vi "Break down String.vi"(6 "PlayerID":u8=1, 8 "Error in":errorcluster, 11 "Input String":string) -> (0 "Error Out":errorcluster, 3 "Output":string[](array[string]))   [LabVIEW 2018, in "Vires VTD System Explorer.lvlib"]
uses:
  Vires VTD System Explorer.lvlib
  <vilib>/regexp/Match Regular Expression.xnode
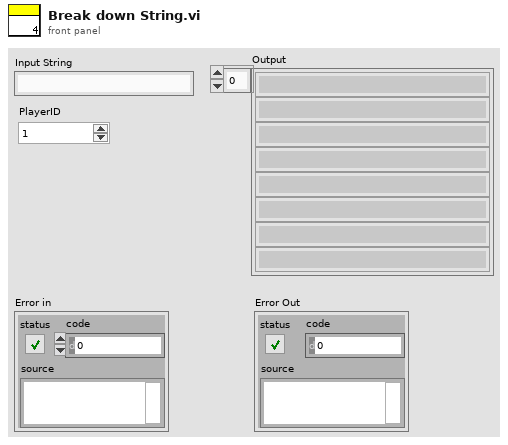
[diagram p1: front panel]
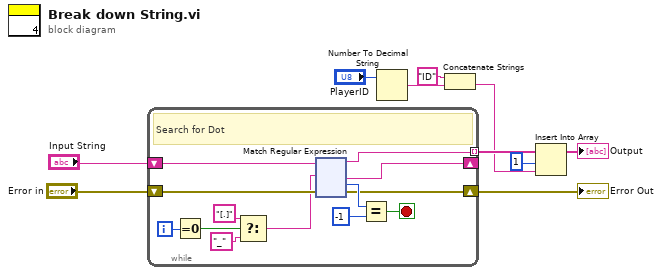
[diagram p0: block diagram]
diagram:
  n1 = while {
    shift-right: [w22] -> _
    shift-left: "Input String" -> [w23]
    tunnel: [w21] -> w4 mode=indexing
    shift-right: [w16] -> w8
    shift-left: "Error in" -> [w17]
    i -> [w15]
    stop <- w18 stop-if-true
    # "Search for Dot"
    n2 = Equal To 0?(x=w15) -> (x = 0?=w14:bool)
    n3 = Select(t="[.]" ("regular expression"), s=w14, f="_" ("regular expression")) -> (s? t:f=w11:string)
    n4 = xnode "Match Regular Expression"("input string"=w23, "regular expression"=w11, "error in"=w17) -> ("before match"=w21:string, "after match"=w22:string, "offset past match"=w20:i32, "error out"=w16:errorcluster)  [unwired: 3 in, 1 out]
    n5 = Equal?(x=w20, y=-1) -> (x = y?=w18:bool)
  }
  "Error Out" <- w8
  n6 = Number To Decimal String(number="PlayerID") -> (decimal integer string=w5:string)  [unwired: 1 in]
  n7 = Concatenate Strings("ID" ("string"), w5) -> (w2:string)
  n8 = Insert Into Array(array=w4, index=1, new element=w2) -> (→"Output":string[])
